vi "高亮.vi"(1 "使能":bool=TRUE, 2 "Y":i32, 3 "X":i32, 4 "进入的数组":bool[][](array[boolean])=[[FALSE]]) -> (0 "输出数组":bool[][](array[boolean]))   [LabVIEW 2017]
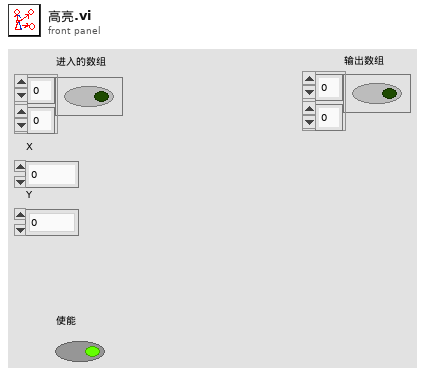
[diagram p1: front panel]
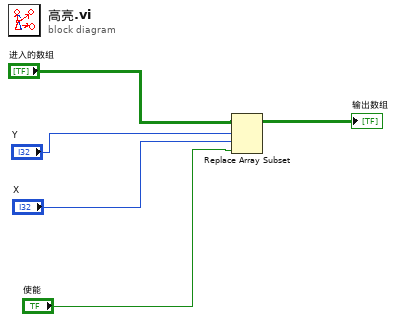
[diagram p0: block diagram]
diagram:
  n1 = Replace Array Subset(array="进入的数组", new element="使能", index (row)="Y", index (col)="X") -> (→"输出数组":bool[][])
